vi "Log Message Fields.vi"(10 "message fields":T1 {"data" format="%x"; "extra" format="%x"; "msgopt" format="%04x"; "msgflag" format="%04x"; "bus" items=["BUSA", "BUSB", "BUSNONE"]; "cwd1" format="%04x"; "cwd2" format="%04x"; "swd1" format="%04x"; "swd2" format="%04x"}, 11 "log file":path=path "c:/ni-rt/VeriStand/Custom Devices/Message Fields.txt") -> ()   [LabVIEW 2020]
uses:
  <instrlib>/BTI1553Lib/Public/Controls/1553 Message Fields.ctl
  <instrlib>/BTI1553Lib/BTI1553LV.lvlib
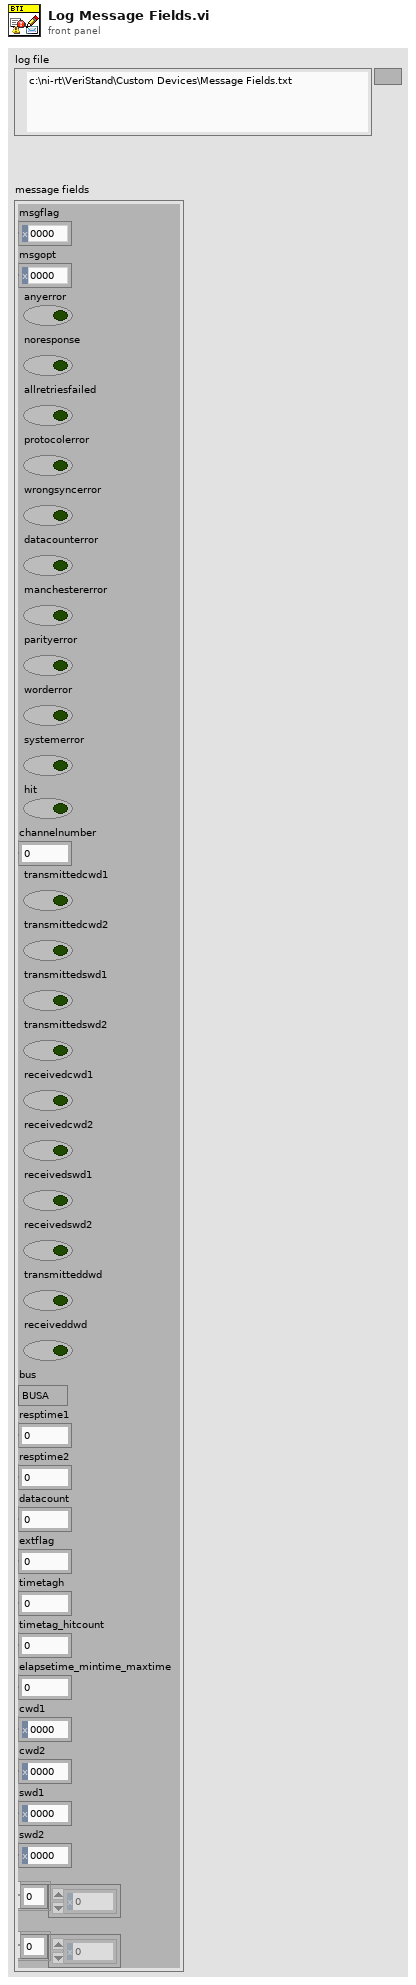
[diagram p1: front panel]
types:
  T1 = typedef "BTI1553LV.lvlib/1553 Message Fields.ctl" = cluster{"msgflag":u16, "msgopt":u16, "anyerror":bool, "noresponse":bool, "allretriesfailed":bool, "protocolerror":bool, "wrongsyncerror":bool, "datacounterror":bool, "manchestererror":bool, "parityerror":bool, "worderror":bool, "systemerror":bool, "hit":bool, "reserved":u8, "channelnumber":i32, "transmittedcwd1":bool, "transmittedcwd2":bool, "transmittedswd1":bool, "transmittedswd2":bool, "receivedcwd1":bool, "receivedcwd2":bool, "receivedswd1":bool, "receivedswd2":bool, "transmitteddwd":bool, "receiveddwd":bool, "reserved":i8, "reserved":i8, "bus":u32, "resptime1":u16, "resptime2":u16, "datacount":u16, "extflag":u16, "timetagh":u32, "timetag_hitcount":u32, "elapsetime_mintime_maxtime":u32, "cwd1":u16, "cwd2":u16, "swd1":u16, "swd2":u16, "data":u16[], "extra":u16[]}
  T2 = cluster{"msgflag":u16, "msgopt":u16, "anyerror":bool, "noresponse":bool, "allretriesfailed":bool, "protocolerror":bool, "wrongsyncerror":bool, "datacounterror":bool, "manchestererror":bool, "parityerror":bool, "worderror":bool, "systemerror":bool, "hit":bool, "reserved":u8, "channelnumber":i32, "transmittedcwd1":bool, "transmittedcwd2":bool, "transmittedswd1":bool, "transmittedswd2":bool, "receivedcwd1":bool, "receivedcwd2":bool, "receivedswd1":bool, "receivedswd2":bool, "transmitteddwd":bool, "receiveddwd":bool, "reserved_1":i8, "reserved_2":i8, "bus":u32, "resptime1":u16, "resptime2":u16, "datacount":u16, "extflag":u16, "timetagh":u32, "timetag_hitcount":u32, "elapsetime_mintime_maxtime":u32, "cwd1":u16, "cwd2":u16, "swd1":u16, "swd2":u16, "data":u16[], "extra":u16[]}
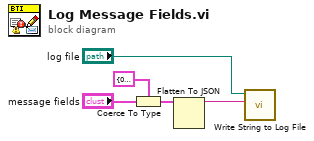
[diagram p0: block diagram]
diagram:
  n1 = Coerce To Type(0:"message fields", 1:T2 {"msgflag"=0, "msgopt"=0, "anyerror"=TRUE, "noresponse"=TRUE, "allretriesfailed"=TRUE, "protocolerror"=FALSE, "wrongsyncerror"=FALSE, "datacounterror"=FALSE, "manchestererror"=FALSE, "parityerror"=FALSE, "worderror"=FALSE, "systemerror"=FALSE, "hit"=FALSE, "reserved"=0, "channelnumber"=0, "transmittedcwd1"=FALSE, "transmittedcwd2"=FALSE, "transmittedswd1"=FALSE, "transmittedswd2"=FALSE, "receivedcwd1"=FALSE, "receivedcwd2"=FALSE, "receivedswd1"=FALSE, "receivedswd2"=FALSE, "transmitteddwd"=FALSE, "receiveddwd"=FALSE, "reserved_1"=0, "reserved_2"=0, "bus"=0, "resptime1"=0, "resptime2"=0, "datacount"=0, "extflag"=0, "timetagh"=0, "timetag_hitcount"=0, "elapsetime_mintime_maxtime"=0, "cwd1"=0, "cwd2"=0, "swd1"=0, "swd2"=0, "data"=[], "extra"=[]} ("message fields")) -> (2:w2:T2)
  n2 = Flatten To JSON(anything=w2) -> (JSON string=w1:string)  [unwired: 2 in, 1 out]
  n3 = call "Write String to Log File.vi"("string to log"=w1, "log file"="log file") -> ()  [unwired: 9 in, 1 out]
